vi "FTW-JSON-Variant-Traverse.vi"(0 "Variant":variant, 1 "Options":T2={"Include Name"=FALSE, "Indent"=0, "Spaces"=4, "Pretty Print"=FALSE, "Real Format"="%#_15g", "Timestamp Format"="%^<%Y-%m-%dT%H:%M:%S%3uZ>T"}, 5 "Type":T1, 7 "Name":string, 11 "error in":errorcluster) -> (4 "JSON String":string, 15 "error out":errorcluster)   [LabVIEW 2015]
uses:
  FTW-JSON-SerializeOptions.ctl
  <vilib>/Utility/Data Type/Type Definitions/Data Type.ctl
  <vilib>/Utility/Data Type/NI_Data Type.lvlib
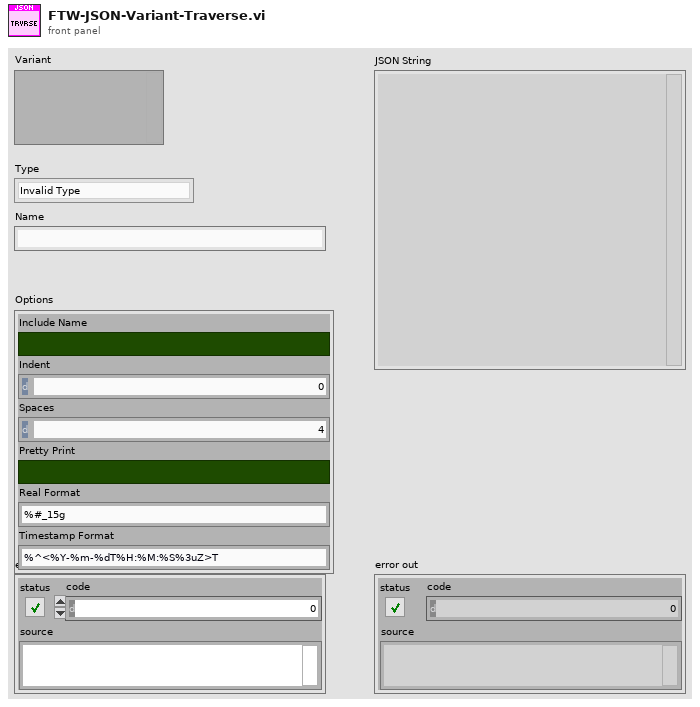
[diagram p1: front panel]
types:
  T1 = typedef "NI_Data Type.lvlib/Data Type.ctl" = enum8{"Invalid Type", "Void", "I8", "I16", "I32", "I64", "U8", "U16", "U32", "U64", "Single Float", "Double Float", "Extended Float", "Single Complex", "Double Complex", "Extended Complex", "Enum U8", "Enum U16", "Enum U32", "Enum U64", "Single Float With Unit", "Double Float With Unit", "Extended Float With Unit", "Single Complex with Unit", "Double Complex with Unit", "Extended Complex with Unit", "Boolean", "String", "Path", "Picture", "Tag", "Array", "Cluster", "Variant", "LV Variant", "Waveform", "Timestamp", "Digital Waveform", "Digital Data", "ExpressData", "Refnum", "External Data", "VI", "Poly VI", "LabVIEW Class Instance", "Fixed Point"}
  T2 = typedef "FTW-JSON-SerializeOptions.ctl" = cluster{"Include Name":bool, "Indent":i32, "Spaces":i32, "Pretty Print":bool, "Real Format":string, "Timestamp Format":string}
  T3 = typedef "NI_Data Type.lvlib/Refnum Type.ctl" = enum16{"NotARefnum", "UnknownRefnum", "Generic", "Datalog", "ByteStream", "Device", "Occurence", "TCPNetConnection", "Auto", "Menu", "Imaq", "Hardware", "DataSocket", "Visa", "IVI", "UDPNetConnection", "Notifier", "Queue", "Irda", "EventReg", "DotNet", "UserEvent", "Callback", "UNUSED_EMPTY_POSITION", "BlueToothNetConnection", "LVObjApp", "LVObjVI", "LVObjUnknown", "GenericClass", "UserDefinedRefnumTag", "DataValue", "RT FIFO", "TDMS File"}
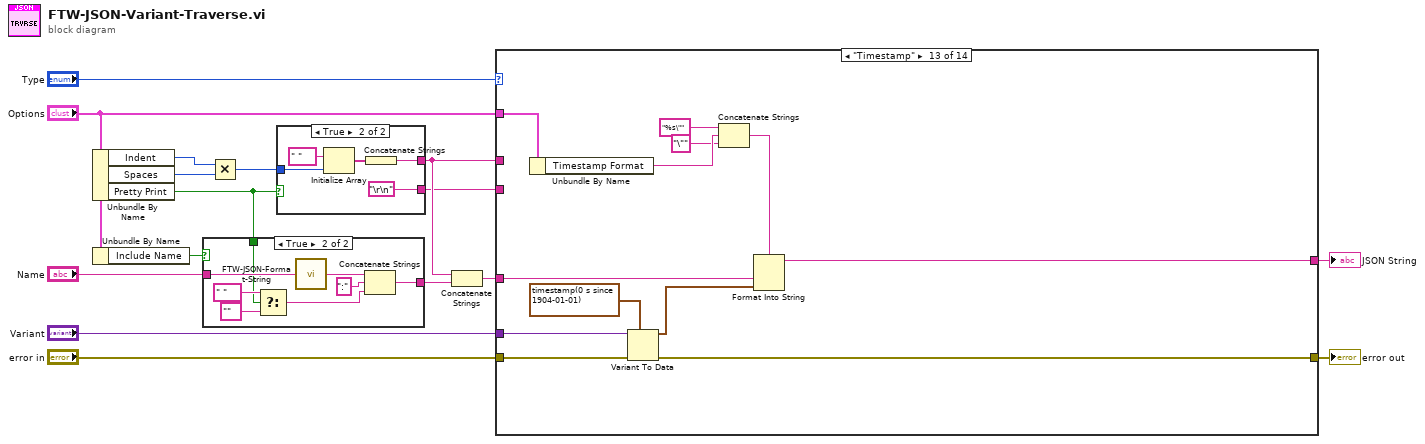
[diagram p0: block diagram]
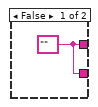
[diagram p2: hidden frame]
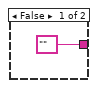
[diagram p3: hidden frame]
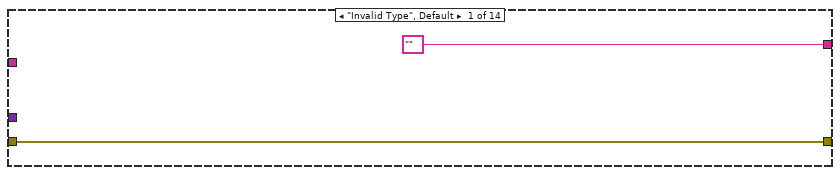
[diagram p4: hidden frame]
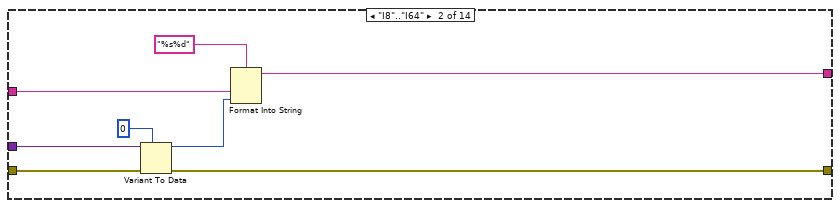
[diagram p5: hidden frame]
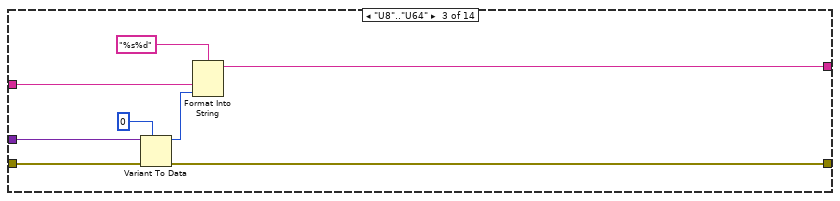
[diagram p6: hidden frame]
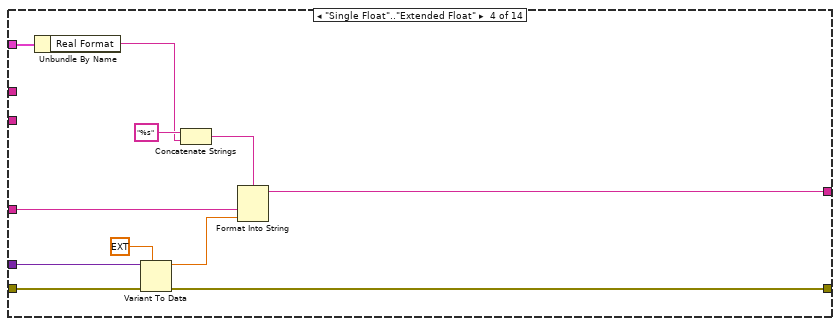
[diagram p7: hidden frame]
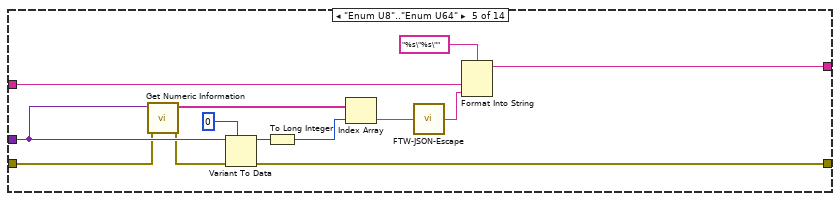
[diagram p8: hidden frame]
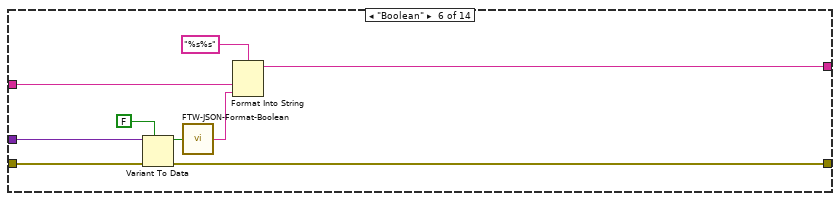
[diagram p9: hidden frame]
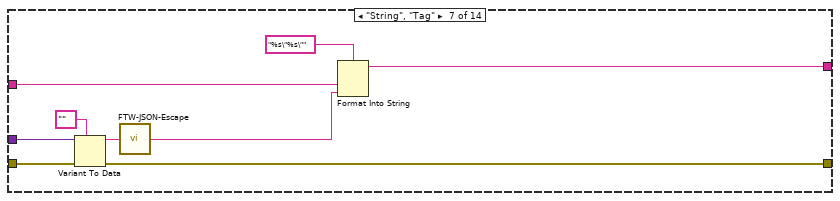
[diagram p10: hidden frame]
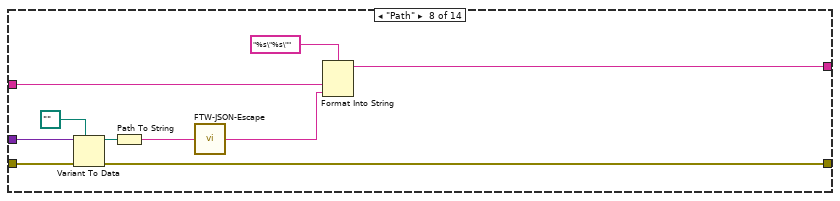
[diagram p11: hidden frame]
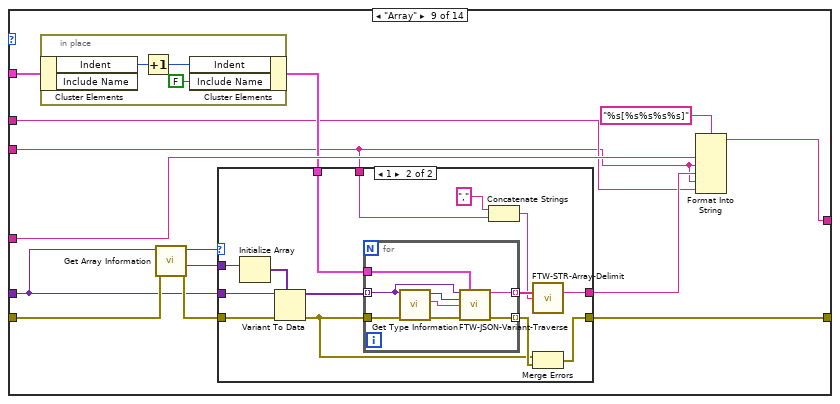
[diagram p12: hidden frame]
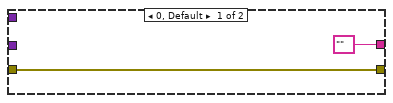
[diagram p13: hidden frame]
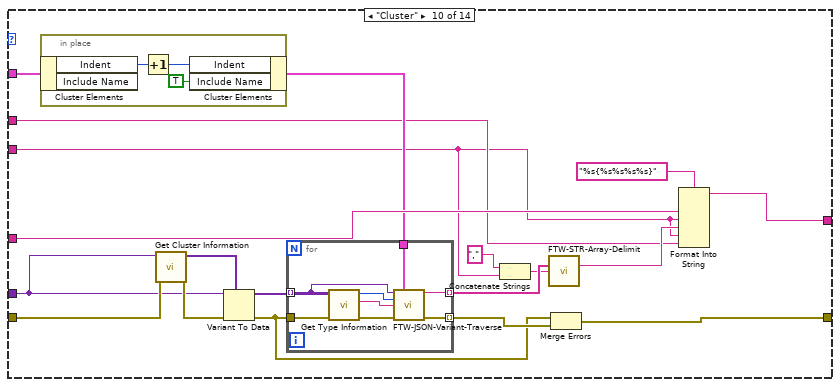
[diagram p14: hidden frame]
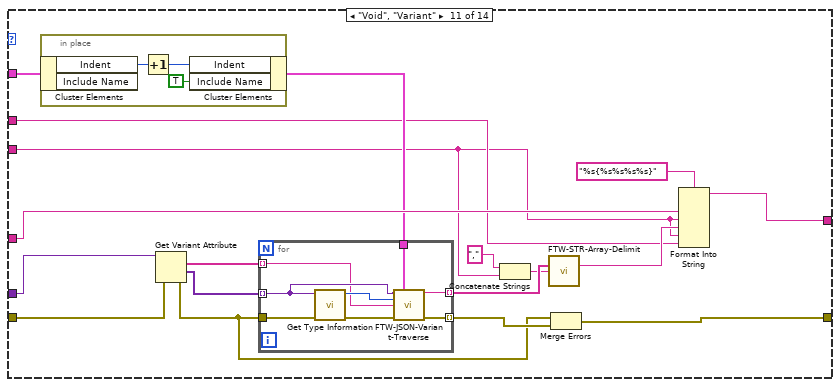
[diagram p15: hidden frame]
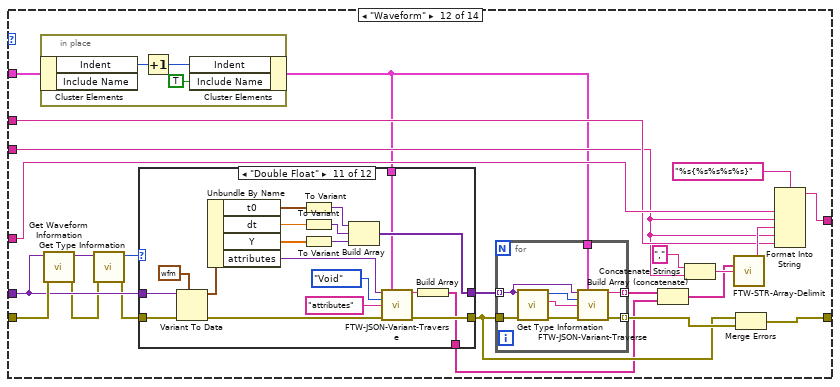
[diagram p16: hidden frame]
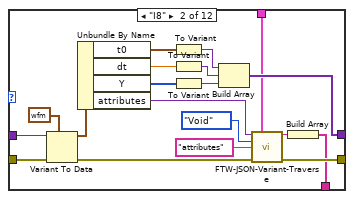
[diagram p18: hidden frame]
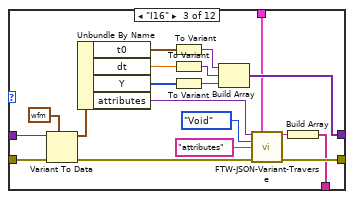
[diagram p19: hidden frame]
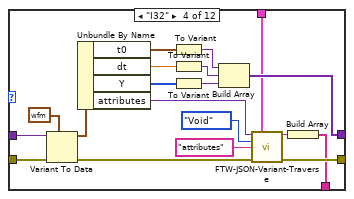
[diagram p20: hidden frame]
diagram:
  n1 = Unbundle By Name("Options") -> ("Indent"=w7:i32, "Spaces"=w9:i32, "Pretty Print"=w1:bool)
  n2 = Unbundle By Name("Options") -> ("Include Name"=w5:bool)
  n3 = case shown="True" w5 {
    tunnel: "Name" -> [_ w22]
    tunnel: ["" ("empty string") w25] -> w12
    tunnel: w1 -> [_ w19]
    frame False {
    }
    frame True {
      n4 = Select(t=" " ("empty string"), s=w19, f="" ("empty string")) -> (s? t:f=w18:string)
      n5 = call "FTW-JSON-Format-String.vi"("LabVIEW String"=w22) -> ("JSON String"=w23:string)
      n6 = Concatenate Strings(w23, ":" ("string"), w18) -> (w25:string)
    }
  }
  n7 = Multiply(x=w7, y=w9) -> (x*y=w8:i32)
  n8 = case shown="True" w1 {
    tunnel: w8 -> [_ w31]
    tunnel: [w26 w29] -> w6
    tunnel: [w26 "\r\n"] -> w4
    frame False {
      w26 = "" ("empty string")
    }
    frame True {
      n9 = Initialize Array(" " ("empty string"), w31) -> (w30:string[])
      n10 = Concatenate Strings(w30) -> (w29:string)
    }
  }
  n11 = Concatenate Strings(w6, w12) -> (w11:string)
  n12 = case shown="\"Timestamp\"" "Type" {
    tunnel: w11 -> [_ w36 w44 w55 w70 w75 w86 w96 w106 w155 w184 w218 w452 w463]
    tunnel: "error in" -> [w33 w41 w49 w60 w62 w82 w91 w101 w114 w161 w190 w224 w457 w462]
    tunnel: [w33 w40 w48 w59 w73 w81 w90 w100 w115 w153 w182 w216 w456 w465] -> w15
    tunnel: ["" ("empty string") w37 w45 w56 w71 w77 w87 w97 w108 w154 w183 w217 w453 w464] -> w14
    tunnel: "Variant" -> [_ w39 w47 w58 w63 w80 w89 w99 w110 w149 w181 w214 w455 w460]
    tunnel: "Options" -> [_ _ _ w52 _ _ _ _ w105 w147 w180 w212 w450 _]
    tunnel: w6 -> [_ _ _ _ _ _ _ _ w103 w144 w177 w210 _ _]
    tunnel: w4 -> [_ _ _ _ _ _ _ _ w102 w143 w176 w209 _ _]
    frame "Invalid Type", Default {
    }
    frame "I8".."I64" {
      n13 = Variant To Data(error in=w41, type=i64 0, Variant=w39) -> (data=w35:i64, error out=w40:errorcluster)
      n14 = Format Into String(format string="%s%d", w36, w35) -> (resulting string=w37:string)  [unwired: 2 in, 1 out]
    }
    frame "U8".."U64" {
      n15 = Variant To Data(error in=w49, type=u64 0, Variant=w47) -> (data=w43:u64, error out=w48:errorcluster)
      n16 = Format Into String(format string="%s%d", w44, w43) -> (resulting string=w45:string)  [unwired: 2 in, 1 out]
    }
    frame "Single Float".."Extended Float" {
      n17 = Unbundle By Name(w52) -> ("Real Format"=w50:string)
      n18 = Variant To Data(error in=w60, type=ext 0.0, Variant=w58) -> (data=w54:ext, error out=w59:errorcluster)
      n19 = Concatenate Strings("%s" ("format string"), w50) -> (w51:string)
      n20 = Format Into String(format string=w51, w55, w54) -> (resulting string=w56:string)  [unwired: 2 in, 1 out]
    }
    frame "Enum U8".."Enum U64" {
      n21 = call <vilib>:"Get Numeric Information.vi"("error in (no error)"=w62, "Variant"=w63) -> ("error out"=w61:errorcluster, "Enum Names"=w68:string[])  [unwired: 6 in, 2 out]
      n22 = Variant To Data(error in=w61, type=u64 0, Variant=w63) -> (data=w67:u64, error out=w73:errorcluster)
      n23 = To Long Integer(number=w67) -> (32bit integer=w66:i32)
      n24 = Index Array(array=w68, index=w66) -> (element=w65:string)
      n25 = call "FTW-JSON-Escape.vi"("String"=w65) -> ("Escaped UTF-8 String"=w64:string)
      n26 = Format Into String(format string="%s\"%s\"", w70, w64) -> (resulting string=w71:string)  [unwired: 2 in, 1 out]
    }
    frame "Boolean" {
      n27 = Variant To Data(error in=w82, type=FALSE, Variant=w80) -> (data=w74:bool, error out=w81:errorcluster)
      n28 = call "FTW-JSON-Format-Boolean.vi"("LabVIEW Boolean"=w74) -> ("JSON Boolean"=w76:string)
      n29 = Format Into String(format string="%s%s", w75, w76) -> (resulting string=w77:string)  [unwired: 2 in, 1 out]
    }
    frame "String", "Tag" {
      n30 = Variant To Data(error in=w91, type="" ("empty string"), Variant=w89) -> (data=w85:string, error out=w90:errorcluster)
      n31 = call "FTW-JSON-Escape.vi"("String"=w85) -> ("Escaped UTF-8 String"=w83:string)
      n32 = Format Into String(format string="%s\"%s\"", w86, w83) -> (resulting string=w87:string)  [unwired: 2 in, 1 out]
    }
    frame "Path" {
      n33 = Variant To Data(error in=w101, type=path "", Variant=w99) -> (data=w95:path, error out=w100:errorcluster)
      n34 = Path To String(path=w95) -> (string=w92:string)
      n35 = call "FTW-JSON-Escape.vi"("String"=w92) -> ("Escaped UTF-8 String"=w94:string)
      n36 = Format Into String(format string="%s\"%s\"", w96, w94) -> (resulting string=w97:string)  [unwired: 2 in, 1 out]
    }
    frame "Array" {
      n37 = in-place {
        n38 = in-place-cluster #1(w105) -> ("Indent"=w118:i32)  [unwired: 1 out]
        n39 = Increment(x=w118) -> (x+1=w117:i32)
        n40 = in-place-cluster #1("Indent"=w117, "Include Name"=FALSE) -> (w104:T2)
      }
      n41 = call <vilib>:"Get Array Information.vi"("error in (no error)"=w114, "Variant"=w110) -> ("error out"=w113:errorcluster, "Array Element Data Type"=w111:variant, "Number of Dimensions"=w112:i32)  [unwired: 6 in, 1 out]
      n42 = case shown="1" w112 {
        tunnel: [w120 w125] -> w115
        tunnel: w113 -> [w120 w133]
        tunnel: w111 -> [_ w128]
        tunnel: ["" ("empty string") w130] -> w107
        tunnel: w110 -> [_ w129]
        tunnel: w104 -> [_ w123]
        tunnel: w102 -> [_ w121]
        frame 0, Default {
        }
        frame 1 {
          n43 = Initialize Array(w128) -> (w127:variant[])  [unwired: 1 in]
          n44 = Variant To Data(error in=w133, type=w127, Variant=w129) -> (data=w126:variant[], error out=w124:errorcluster)
          n45 = for {
            tunnel: w126 -> [w135] mode=indexing
            tunnel: [w141] -> w132 mode=indexing
            tunnel: w124 -> [w140]
            tunnel: [w142] -> w134 mode=indexing
            tunnel: w123 -> [w139]
            n46 = call <vilib>:"Get Type Information.vi"("error in (no error)"=w140, "Variant"=w135) -> ("error out"=w138:errorcluster, "Name"=w137:string, "Type"=w136:T1)  [unwired: 5 in, 2 out]
            n47 = call "FTW-JSON-Variant-Traverse.vi"("Variant"=w135, "Options"=w139, "Type"=w136, "Name"=w137, "error in"=w138) -> ("JSON String"=w141:string, "error out"=w142:errorcluster)  [unwired: 9 in]
          }
          n48 = Concatenate Strings("," ("Delimiter"), w121) -> (w122:string)
          n49 = call "FTW-STR-Array-Delimit.vi"("Array of Strings"=w132, "Delimiter"=w122) -> ("Delimited String"=w130:string)  [unwired: 13 in]
          n50 = Merge Errors(w124, w134) -> (w125:errorcluster)
        }
      }
      n51 = Format Into String(format string="%s[%s%s%s%s]", w106, w102, w107, w102, w103) -> (resulting string=w108:string)  [unwired: 2 in, 1 out]
    }
    frame "Cluster" {
      n52 = in-place {
        n53 = in-place-cluster #2(w147) -> ("Indent"=w164:i32)  [unwired: 1 out]
        n54 = Increment(x=w164) -> (x+1=w163:i32)
        n55 = in-place-cluster #2("Indent"=w163, "Include Name"=TRUE) -> (w146:T2)
      }
      n56 = call <vilib>:"Get Cluster Information.vi"("error in (no error)"=w161, "Variant"=w149) -> ("error out"=w152:errorcluster, "Cluster Elements"=w150:variant[])  [unwired: 8 in]
      n57 = Variant To Data(error in=w152, type=w150, Variant=w149) -> (data=w148:variant[], error out=w151:errorcluster)
      n58 = for {
        tunnel: w148 -> [w167] mode=indexing
        tunnel: [w170] -> w159 mode=indexing
        tunnel: w151 -> [w172]
        tunnel: [w171] -> w160 mode=indexing
        tunnel: w146 -> [w169]
        n59 = call <vilib>:"Get Type Information.vi"("error in (no error)"=w172, "Variant"=w167) -> ("error out"=w168:errorcluster, "Name"=w165:string, "Type"=w166:T1)  [unwired: 5 in, 2 out]
        n60 = call "FTW-JSON-Variant-Traverse.vi"("Variant"=w167, "Options"=w169, "Type"=w166, "Name"=w165, "error in"=w168) -> ("JSON String"=w170:string, "error out"=w171:errorcluster)  [unwired: 9 in]
      }
      n61 = Concatenate Strings("," ("Delimiter"), w143) -> (w145:string)
      n62 = call "FTW-STR-Array-Delimit.vi"("Array of Strings"=w159, "Delimiter"=w145) -> ("Delimited String"=w157:string)  [unwired: 13 in]
      n63 = Merge Errors(w151, w160) -> (w153:errorcluster)
      n64 = Format Into String(format string="%s{%s%s%s%s}", w155, w143, w157, w143, w144) -> (resulting string=w154:string)  [unwired: 2 in, 1 out]
    }
    frame "Void", "Variant" {
      n65 = in-place {
        n66 = in-place-cluster #3(w180) -> ("Indent"=w193:i32)  [unwired: 1 out]
        n67 = Increment(x=w193) -> (x+1=w192:i32)
        n68 = in-place-cluster #3("Indent"=w192, "Include Name"=TRUE) -> (w179:T2)
      }
      n69 = Get Variant Attribute(Variant=w181, error in=w190) -> (names=w173:string[], values=w174:variant[], error out=w175:errorcluster)  [unwired: 2 in, 1 out]
      n70 = for {
        tunnel: w174 -> [w196] mode=indexing
        tunnel: [w200] -> w188 mode=indexing
        tunnel: w175 -> [w198]
        tunnel: [w201] -> w189 mode=indexing
        tunnel: w179 -> [w199]
        tunnel: w173 -> [w194] mode=indexing
        n71 = call <vilib>:"Get Type Information.vi"("error in (no error)"=w198, "Variant"=w196) -> ("error out"=w197:errorcluster, "Type"=w195:T1)  [unwired: 5 in, 3 out]
        n72 = call "FTW-JSON-Variant-Traverse.vi"("Variant"=w196, "Options"=w199, "Type"=w195, "Name"=w194, "error in"=w197) -> ("JSON String"=w200:string, "error out"=w201:errorcluster)  [unwired: 9 in]
      }
      n73 = Concatenate Strings("," ("Delimiter"), w176) -> (w178:string)
      n74 = call "FTW-STR-Array-Delimit.vi"("Array of Strings"=w188, "Delimiter"=w178) -> ("Delimited String"=w186:string)  [unwired: 13 in]
      n75 = Merge Errors(w175, w189) -> (w182:errorcluster)
      n76 = Format Into String(format string="%s{%s%s%s%s}", w184, w176, w186, w176, w177) -> (resulting string=w183:string)  [unwired: 2 in, 1 out]
    }
    frame "Waveform" {
      n77 = in-place {
        n78 = in-place-cluster #4(w212) -> ("Indent"=w437:i32)  [unwired: 1 out]
        n79 = Increment(x=w437) -> (x+1=w436:i32)
        n80 = in-place-cluster #4("Indent"=w436, "Include Name"=TRUE) -> (w204:T2)
      }
      n81 = call <vilib>:"Get Waveform Information.vi"("error in (no error)"=w224, "Variant"=w214) -> ("error out"=w207:errorcluster, "Y Array Type"=w208:variant)  [unwired: 8 in]
      n82 = call <vilib>:"Get Type Information.vi"("error in (no error)"=w207, "Variant"=w208) -> ("error out"=w206:errorcluster, "Type"=w205:T1)  [unwired: 5 in, 3 out]
      n83 = case shown="\"Double Float\"" w205 {
        tunnel: [w225 w232 w251 w270 w289 w308 w327 w346 w365 w384 w403 w422] -> w215
        tunnel: w214 -> [_ w236 w255 w274 w293 w312 w331 w350 w369 w388 w407 w426]
        tunnel: [_ w244 w263 w282 w301 w320 w339 w358 w377 w396 w415 w434] -> w213
        tunnel: w206 -> [w225 w240 w259 w278 w297 w316 w335 w354 w373 w392 w411 w430]
        tunnel: w204 -> [_ w231 w250 w269 w288 w307 w326 w345 w364 w383 w402 w421]
        tunnel: [_ w226 w245 w264 w283 w302 w321 w340 w359 w378 w397 w416] -> w202
        frame "Invalid Type", Default {
        }
        frame "I8" {
          n84 = Variant To Data(error in=w240, type=waveform(i8) {"t0"=timestamp(0 s since 1904-01-01), "dt"=1.0, "Y"=[]} ("Waveform"), Variant=w236) -> (data=w234:waveform(i8), error out=w233:errorcluster)
          n85 = Unbundle By Name(w234) -> ("t0"=w239:timestamp, "dt"=w238:dbl, "Y"=w237:i8[], "attributes"=w230:variant)
          n86 = To Variant(anything=w239) -> (Variant=w243:variant)
          n87 = To Variant(anything=w238) -> (Variant=w242:variant)
          n88 = To Variant(anything=w237) -> (Variant=w241:variant)
          n89 = Build Array(w243, w242, w241) -> (w244:variant[])
          n90 = call "FTW-JSON-Variant-Traverse.vi"("Variant"=w230, "Options"=w231, "Type"=Data_Type."Void", "Name"="attributes", "error in"=w233) -> ("JSON String"=w227:string, "error out"=w232:errorcluster)  [unwired: 9 in]
          n91 = Build Array(w227) -> (w226:string[])
        }
        frame "I16" {
          n92 = Variant To Data(error in=w259, type=waveform(i16) {"t0"=timestamp(0 s since 1904-01-01), "dt"=1.0, "Y"=[]} ("Waveform"), Variant=w255) -> (data=w253:waveform(i16), error out=w252:errorcluster)
          n93 = Unbundle By Name(w253) -> ("t0"=w258:timestamp, "dt"=w257:dbl, "Y"=w256:i16[], "attributes"=w249:variant)
          n94 = To Variant(anything=w258) -> (Variant=w262:variant)
          n95 = To Variant(anything=w257) -> (Variant=w261:variant)
          n96 = To Variant(anything=w256) -> (Variant=w260:variant)
          n97 = Build Array(w262, w261, w260) -> (w263:variant[])
          n98 = call "FTW-JSON-Variant-Traverse.vi"("Variant"=w249, "Options"=w250, "Type"=Data_Type."Void", "Name"="attributes", "error in"=w252) -> ("JSON String"=w246:string, "error out"=w251:errorcluster)  [unwired: 9 in]
          n99 = Build Array(w246) -> (w245:string[])
        }
        frame "I32" {
          n100 = Variant To Data(error in=w278, type=waveform(i32) {"t0"=timestamp(0 s since 1904-01-01), "dt"=1.0, "Y"=[]} ("Waveform"), Variant=w274) -> (data=w272:waveform(i32), error out=w271:errorcluster)
          n101 = Unbundle By Name(w272) -> ("t0"=w277:timestamp, "dt"=w276:dbl, "Y"=w275:i32[], "attributes"=w268:variant)
          n102 = To Variant(anything=w277) -> (Variant=w281:variant)
          n103 = To Variant(anything=w276) -> (Variant=w280:variant)
          n104 = To Variant(anything=w275) -> (Variant=w279:variant)
          n105 = Build Array(w281, w280, w279) -> (w282:variant[])
          n106 = call "FTW-JSON-Variant-Traverse.vi"("Variant"=w268, "Options"=w269, "Type"=Data_Type."Void", "Name"="attributes", "error in"=w271) -> ("JSON String"=w265:string, "error out"=w270:errorcluster)  [unwired: 9 in]
          n107 = Build Array(w265) -> (w264:string[])
        }
        frame "I64" {
          n108 = Variant To Data(error in=w297, type=waveform(i64) {"t0"=timestamp(0 s since 1904-01-01), "dt"=1.0, "Y"=[]} ("Waveform"), Variant=w293) -> (data=w291:waveform(i64), error out=w290:errorcluster)
          n109 = Unbundle By Name(w291) -> ("t0"=w296:timestamp, "dt"=w295:dbl, "Y"=w294:i64[], "attributes"=w287:variant)
          n110 = To Variant(anything=w296) -> (Variant=w300:variant)
          n111 = To Variant(anything=w295) -> (Variant=w299:variant)
          n112 = To Variant(anything=w294) -> (Variant=w298:variant)
          n113 = Build Array(w300, w299, w298) -> (w301:variant[])
          n114 = call "FTW-JSON-Variant-Traverse.vi"("Variant"=w287, "Options"=w288, "Type"=Data_Type."Void", "Name"="attributes", "error in"=w290) -> ("JSON String"=w284:string, "error out"=w289:errorcluster)  [unwired: 9 in]
          n115 = Build Array(w284) -> (w283:string[])
        }
        frame "U8" {
          n116 = Variant To Data(error in=w316, type=waveform(u8) {"t0"=timestamp(0 s since 1904-01-01), "dt"=1.0, "Y"=[]} ("Waveform"), Variant=w312) -> (data=w310:waveform(u8), error out=w309:errorcluster)
          n117 = Unbundle By Name(w310) -> ("t0"=w315:timestamp, "dt"=w314:dbl, "Y"=w313:u8[], "attributes"=w306:variant)
          n118 = To Variant(anything=w315) -> (Variant=w319:variant)
          n119 = To Variant(anything=w314) -> (Variant=w318:variant)
          n120 = To Variant(anything=w313) -> (Variant=w317:variant)
          n121 = Build Array(w319, w318, w317) -> (w320:variant[])
          n122 = call "FTW-JSON-Variant-Traverse.vi"("Variant"=w306, "Options"=w307, "Type"=Data_Type."Void", "Name"="attributes", "error in"=w309) -> ("JSON String"=w303:string, "error out"=w308:errorcluster)  [unwired: 9 in]
          n123 = Build Array(w303) -> (w302:string[])
        }
        frame "U16" {
          n124 = Variant To Data(error in=w335, type=waveform(u16) {"t0"=timestamp(0 s since 1904-01-01), "dt"=1.0, "Y"=[]} ("Waveform"), Variant=w331) -> (data=w329:waveform(u16), error out=w328:errorcluster)
          n125 = Unbundle By Name(w329) -> ("t0"=w334:timestamp, "dt"=w333:dbl, "Y"=w332:u16[], "attributes"=w325:variant)
          n126 = To Variant(anything=w334) -> (Variant=w338:variant)
          n127 = To Variant(anything=w333) -> (Variant=w337:variant)
          n128 = To Variant(anything=w332) -> (Variant=w336:variant)
          n129 = Build Array(w338, w337, w336) -> (w339:variant[])
          n130 = call "FTW-JSON-Variant-Traverse.vi"("Variant"=w325, "Options"=w326, "Type"=Data_Type."Void", "Name"="attributes", "error in"=w328) -> ("JSON String"=w322:string, "error out"=w327:errorcluster)  [unwired: 9 in]
          n131 = Build Array(w322) -> (w321:string[])
        }
        frame "U32" {
          n132 = Variant To Data(error in=w354, type=waveform(u32) {"t0"=timestamp(0 s since 1904-01-01), "dt"=1.0, "Y"=[]} ("Waveform"), Variant=w350) -> (data=w348:waveform(u32), error out=w347:errorcluster)
          n133 = Unbundle By Name(w348) -> ("t0"=w353:timestamp, "dt"=w352:dbl, "Y"=w351:u32[], "attributes"=w344:variant)
          n134 = To Variant(anything=w353) -> (Variant=w357:variant)
          n135 = To Variant(anything=w352) -> (Variant=w356:variant)
          n136 = To Variant(anything=w351) -> (Variant=w355:variant)
          n137 = Build Array(w357, w356, w355) -> (w358:variant[])
          n138 = call "FTW-JSON-Variant-Traverse.vi"("Variant"=w344, "Options"=w345, "Type"=Data_Type."Void", "Name"="attributes", "error in"=w347) -> ("JSON String"=w341:string, "error out"=w346:errorcluster)  [unwired: 9 in]
          n139 = Build Array(w341) -> (w340:string[])
        }
        frame "U64" {
          n140 = Variant To Data(error in=w373, type=waveform(u64) {"t0"=timestamp(0 s since 1904-01-01), "dt"=1.0, "Y"=[]} ("Waveform"), Variant=w369) -> (data=w367:waveform(u64), error out=w366:errorcluster)
          n141 = Unbundle By Name(w367) -> ("t0"=w372:timestamp, "dt"=w371:dbl, "Y"=w370:u64[], "attributes"=w363:variant)
          n142 = To Variant(anything=w372) -> (Variant=w376:variant)
          n143 = To Variant(anything=w371) -> (Variant=w375:variant)
          n144 = To Variant(anything=w370) -> (Variant=w374:variant)
          n145 = Build Array(w376, w375, w374) -> (w377:variant[])
          n146 = call "FTW-JSON-Variant-Traverse.vi"("Variant"=w363, "Options"=w364, "Type"=Data_Type."Void", "Name"="attributes", "error in"=w366) -> ("JSON String"=w360:string, "error out"=w365:errorcluster)  [unwired: 9 in]
          n147 = Build Array(w360) -> (w359:string[])
        }
        frame "Single Float" {
          n148 = Variant To Data(error in=w392, type=waveform(sgl) {"t0"=timestamp(0 s since 1904-01-01), "dt"=1.0, "Y"=[]} ("Waveform"), Variant=w388) -> (data=w386:waveform(sgl), error out=w385:errorcluster)
          n149 = Unbundle By Name(w386) -> ("t0"=w391:timestamp, "dt"=w390:dbl, "Y"=w389:sgl[], "attributes"=w382:variant)
          n150 = To Variant(anything=w391) -> (Variant=w395:variant)
          n151 = To Variant(anything=w390) -> (Variant=w394:variant)
          n152 = To Variant(anything=w389) -> (Variant=w393:variant)
          n153 = Build Array(w395, w394, w393) -> (w396:variant[])
          n154 = call "FTW-JSON-Variant-Traverse.vi"("Variant"=w382, "Options"=w383, "Type"=Data_Type."Void", "Name"="attributes", "error in"=w385) -> ("JSON String"=w379:string, "error out"=w384:errorcluster)  [unwired: 9 in]
          n155 = Build Array(w379) -> (w378:string[])
        }
        frame "Double Float" {
          n156 = Variant To Data(error in=w411, type=waveform(dbl) {"t0"=timestamp(0 s since 1904-01-01), "dt"=1.0, "Y"=[]} ("Waveform"), Variant=w407) -> (data=w405:waveform(dbl), error out=w404:errorcluster)
          n157 = Unbundle By Name(w405) -> ("t0"=w410:timestamp, "dt"=w409:dbl, "Y"=w408:dbl[], "attributes"=w401:variant)
          n158 = To Variant(anything=w410) -> (Variant=w414:variant)
          n159 = To Variant(anything=w409) -> (Variant=w413:variant)
          n160 = To Variant(anything=w408) -> (Variant=w412:variant)
          n161 = Build Array(w414, w413, w412) -> (w415:variant[])
          n162 = call "FTW-JSON-Variant-Traverse.vi"("Variant"=w401, "Options"=w402, "Type"=Data_Type."Void", "Name"="attributes", "error in"=w404) -> ("JSON String"=w398:string, "error out"=w403:errorcluster)  [unwired: 9 in]
          n163 = Build Array(w398) -> (w397:string[])
        }
        frame "Extended Float" {
          n164 = Variant To Data(error in=w430, type=waveform(ext) {"t0"=timestamp(0 s since 1904-01-01), "dt"=1.0, "Y"=[]} ("Waveform"), Variant=w426) -> (data=w424:waveform(ext), error out=w423:errorcluster)
          n165 = Unbundle By Name(w424) -> ("t0"=w429:timestamp, "dt"=w428:dbl, "Y"=w427:ext[], "attributes"=w420:variant)
          n166 = To Variant(anything=w429) -> (Variant=w433:variant)
          n167 = To Variant(anything=w428) -> (Variant=w432:variant)
          n168 = To Variant(anything=w427) -> (Variant=w431:variant)
          n169 = Build Array(w433, w432, w431) -> (w434:variant[])
          n170 = call "FTW-JSON-Variant-Traverse.vi"("Variant"=w420, "Options"=w421, "Type"=Data_Type."Void", "Name"="attributes", "error in"=w423) -> ("JSON String"=w417:string, "error out"=w422:errorcluster)  [unwired: 9 in]
          n171 = Build Array(w417) -> (w416:string[])
        }
      }
      n172 = for {
        tunnel: w213 -> [w440] mode=indexing
        tunnel: [w443] -> w222 mode=indexing
        tunnel: w215 -> [w445]
        tunnel: [w444] -> w223 mode=indexing
        tunnel: w204 -> [w442]
        n173 = call <vilib>:"Get Type Information.vi"("error in (no error)"=w445, "Variant"=w440) -> ("error out"=w441:errorcluster, "Name"=w438:string, "Type"=w439:T1)  [unwired: 5 in, 2 out]
        n174 = call "FTW-JSON-Variant-Traverse.vi"("Variant"=w440, "Options"=w442, "Type"=w439, "Name"=w438, "error in"=w441) -> ("JSON String"=w443:string, "error out"=w444:errorcluster)  [unwired: 9 in]
      }
      n175 = Build Array (concatenate)(w222, w202) -> (w203:string[])
      n176 = Concatenate Strings("," ("Delimiter"), w209) -> (w211:string)
      n177 = call "FTW-STR-Array-Delimit.vi"("Array of Strings"=w203, "Delimiter"=w211) -> ("Delimited String"=w220:string)  [unwired: 13 in]
      n178 = Merge Errors(w215, w223) -> (w216:errorcluster)
      n179 = Format Into String(format string="%s{%s%s%s%s}", w218, w209, w220, w209, w210) -> (resulting string=w217:string)  [unwired: 2 in, 1 out]
    }
    frame "Timestamp" {
      n180 = Unbundle By Name(w450) -> ("Timestamp Format"=w447:string)
      n181 = Variant To Data(error in=w457, type=timestamp(0 s since 1904-01-01), Variant=w455) -> (data=w449:timestamp, error out=w456:errorcluster)
      n182 = Concatenate Strings("%s\"" ("format string"), w447, "\"" ("string")) -> (w448:string)
      n183 = Format Into String(format string=w448, w452, w449) -> (resulting string=w453:string)  [unwired: 2 in, 1 out]
    }
    frame "Refnum" {
      n184 = call <vilib>:"Get Refnum Information.vi"("error in (no error)"=w462, "Variant"=w460) -> ("error out"=w461:errorcluster, "Strict Type"=w458:variant, "Reference Type"=w459:T3)  [unwired: 6 in, 1 out]
      n185 = case shown="\"NotARefnum\", Default" w459 {
        tunnel: [w467 w470 w484] -> w465
        tunnel: ["" ("empty string") w474 w482] -> w464
        tunnel: w463 -> [_ w473 w481]
        tunnel: w461 -> [w467 w470 w477]
        tunnel: w460 -> [_ w469 w476]
        tunnel: w458 -> [_ _ _]
        frame "NotARefnum", Default {
        }
        frame "ByteStream".."TCPNetConnection", "UDPNetConnection".."Queue", "EventReg".."UserEvent", "DataValue".."TDMS File" {
          n186 = Variant To Flattened String(Variant=w469) -> (data string=w468:string)  [unwired: 1 out]
          n187 = Type Cast(type=u32 0 ("empty string"), x=w468) -> (*(type *) &x=w471:u32)
          n188 = Format Into String(format string="%s%d", w473, w471) -> (resulting string=w474:string)  [unwired: 2 in, 1 out]
        }
        frame "Visa", "UserDefinedRefnumTag" {
          n189 = Variant To Data(error in=w477, type="" ("empty string"), Variant=w476) -> (data=w480:string, error out=w484:errorcluster)
          n190 = call "FTW-JSON-Escape.vi"("String"=w480) -> ("Escaped UTF-8 String"=w478:string)
          n191 = Format Into String(format string="%s\"%s\"", w481, w478) -> (resulting string=w482:string)  [unwired: 2 in, 1 out]
        }
      }
    }
  }
  "error out" <- w15
  "JSON String" <- w14
